vi "TestBench.Tester.vi"() -> ()   [LabVIEW 2015]
uses:
  TestBenchVariables.vi
panel:
  in  "Reset":bool
  in  "stop":bool
  out "Error":errorcluster
  out "Unconfirmed Error?":bool
  out "Voltage PV":dbl(knob) scale=0.0..5.0
  out "Current PV [mA]":dbl(knob) scale=0.0..200.0
  out "RPM PV":dbl(knob) scale=0.0..500.0
  in  "Serwo Angle SP":dbl(knob) scale=0.0..180.0
  in  "Motor Enable?":bool
  in  "Voltage SP":dbl(slide) scale=0.0..5.0
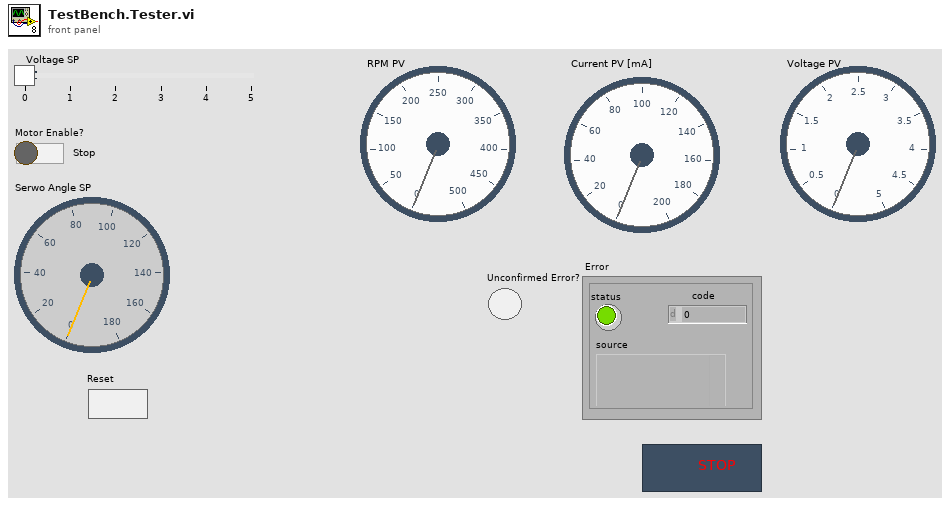
[diagram p1: front panel]
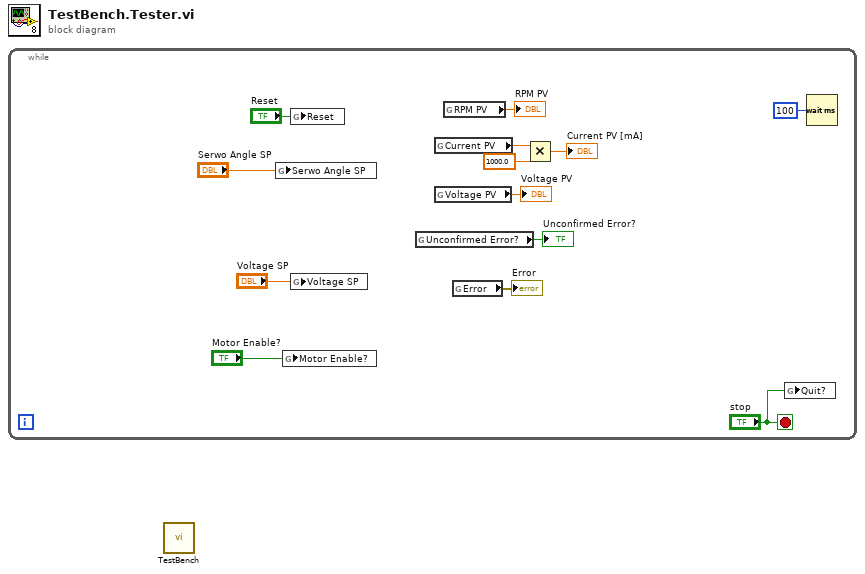
[diagram p0: block diagram]
diagram:
  n1 = while {
    stop <- "stop" stop-if-true
    n2 = global write "TestBenchVariables.vi" "Serwo Angle SP"("Serwo Angle SP") -> ()
    n3 = global write "TestBenchVariables.vi" "Motor Enable?"("Motor Enable?") -> ()
    n4 = global write "TestBenchVariables.vi" "Reset"("Reset") -> ()
    n5 = global write "TestBenchVariables.vi" "Voltage SP"("Voltage SP") -> ()
    n6 = global read "TestBenchVariables.vi" "Unconfirmed Error?"() -> (→"Unconfirmed Error?":bool)
    n7 = global read "TestBenchVariables.vi" "Current PV"() -> (w3:dbl)
    n8 = global read "TestBenchVariables.vi" "Voltage PV"() -> (→"Voltage PV":dbl)
    n9 = global read "TestBenchVariables.vi" "RPM PV"() -> (→"RPM PV":dbl)
    n10 = global read "TestBenchVariables.vi" "Error"() -> (→"Error":errorcluster)
    n11 = Multiply(x=w3, y=1000.0) -> (x*y=→"Current PV [mA]":dbl)
    n12 = global write "TestBenchVariables.vi" "Quit?"("stop") -> ()
    n13 = Wait (ms)(milliseconds to wait=u32 100) -> ()  [unwired: 1 out]
  }
  n14 = call "TestBench.vi"() -> ()  [unwired: 12 in]
